vi "TMP Comms.vi"() -> ()   [LabVIEW 2023]
panel:
  out "error out":errorcluster
  out "read buffer":string
  in  "VISA resource name":refnum<visa-resource-name>
  out "concatenated string":string
  in  "Command":string
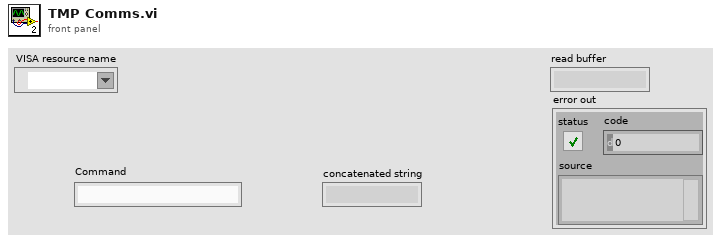
[diagram p1: front panel]
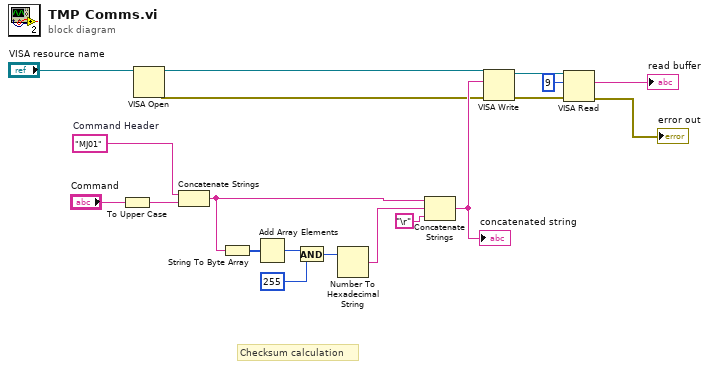
[diagram p0: block diagram]
diagram:
  w17 = "MJ01"  # Command Header
  # "Checksum calculation"
  n1 = To Upper Case(1:"Command") -> (0:w18:string)
  n2 = VISA Open(VISA resource name="VISA resource name") -> (VISA resource name=w7:refnum<visa-resource-name>, error out=w8:errorcluster)  [unwired: 4 in]
  n3 = Concatenate Strings(w17, w18) -> (w12:string)
  n4 = String To Byte Array(string=w12) -> (unsigned byte array=w16:u8[])
  n5 = Add Array Elements(numeric array=w16) -> (sum=w15:u8)
  n6 = And(x=w15, y=u8 255) -> (x .and. y?=w13:u8)
  n7 = Number To Hexadecimal String(2:w13) -> (0:w11:string)  [unwired: 1 in]
  n8 = Concatenate Strings(w12, w11, "\r") -> (w9:string)
  "concatenated string" <- w9
  n9 = VISA Write(VISA resource name=w7, write buffer=w9, error in (no error)=w8) -> (VISA resource name out=w6:refnum<visa-resource-name>, error out=w5:errorcluster)  [unwired: 1 out]
  n10 = VISA Read(VISA resource name=w6, byte count=u32 9, error in (no error)=w5) -> (read buffer=→"read buffer":string, error out=→"error out":errorcluster)  [unwired: 2 out]
